vi "initialize.vi"(8 "error in (no error)":errorcluster, 11 "S4ICS in":refnum<class "S4ICS.lvclass">) -> (0 "error out":errorcluster, 3 "S4ICS out":refnum<class "S4ICS.lvclass">)   [LabVIEW 2018, in "S4ICS.lvclass"]
uses:
  S4ICS.lvclass
  S4ICS.lvclass/S4ICS.ctl
  RxTx/RxTx.lvclass
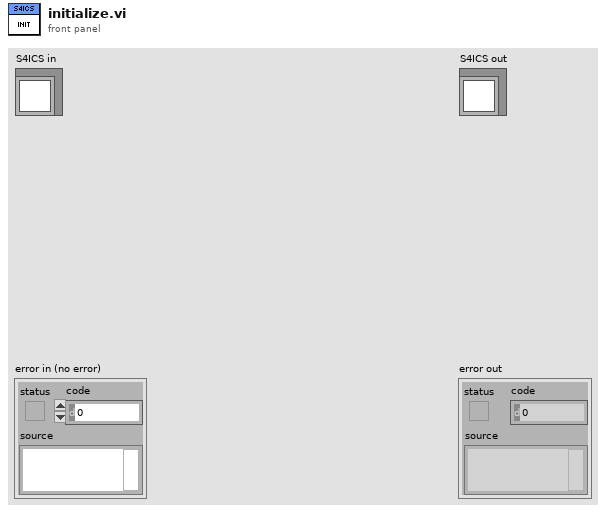
[diagram p1: front panel]
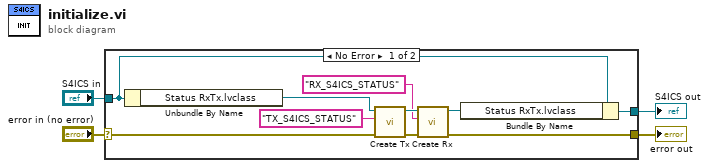
[diagram p0: block diagram]
diagram:
  n1 = case shown="No Error" "error in (no error)" {
    selector: "error in (no error)" -> [w9 w16]
    tunnel: [w6 w16] -> w3
    tunnel: [w5 w15] -> w1
    tunnel: "S4ICS in" -> [w14 w15]
    frame No Error {
      n2 = Unbundle By Name(w14) -> ("Status RxTx.lvclass"=w13:refnum<class "RxTx.lvclass">)
      n3 = call "Create Tx.vi"("error in (no error)"=w9, "Writer Name"="TX_S4ICS_STATUS", "RxTx in"=w13) -> ("error out"=w10:errorcluster, "RxTx out"=w12:refnum<class "RxTx.lvclass">)  [unwired: 7 in]
      n4 = call "Create Rx.vi"("error in (no error)"=w10, "Reader Name"="RX_S4ICS_STATUS" ("Writer Name"), "RxTx in"=w12) -> ("error out"=w6:errorcluster, "RxTx out"=w11:refnum<class "RxTx.lvclass">)  [unwired: 7 in]
      n5 = Bundle By Name(cluster=w14, "Status RxTx.lvclass"=w11) -> (w5:refnum<class "S4ICS.lvclass">)
    }
    frame Error {
    }
  }
  "error out" <- w3
  "S4ICS out" <- w1
